vi "ChannelNamingExample.vi"() -> ()   [LabVIEW 2023]
uses:
  <vilib>/DAQmx/read.llb/DAQmx Read (Analog 1D Wfm NChan NSamp).vi
  <vilib>/DAQmx/create/channels.llb/DAQmx Create Channel (AI-Voltage-Basic).vi
  <vilib>/DAQmx/configure/timing.llb/DAQmx Timing (Sample Clock).vi
  <vilib>/DAQmx/miscellaneous.llb/DAQmx Fill In Error Info.vi
panel:
  out "data":waveform(dbl)[](array[waveform])
  out "Waveform Chart":waveform(dbl)[](graph)
  in  "Stop":bool
  in  "Channel Names":string[](array[string])
  in  "Input Channels":tag
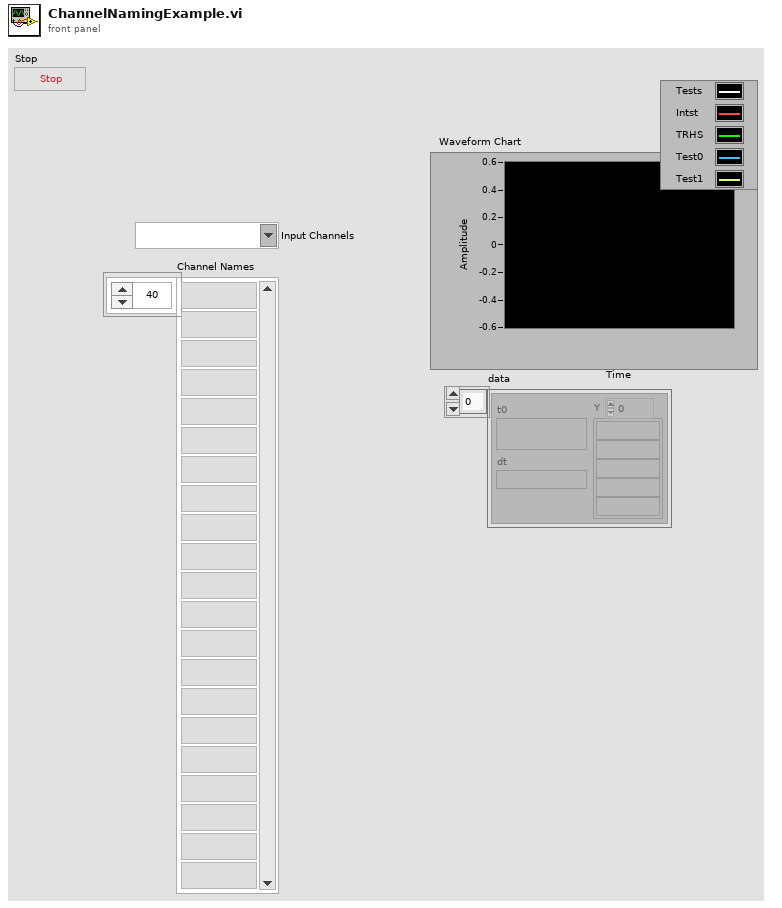
[diagram p1: front panel]
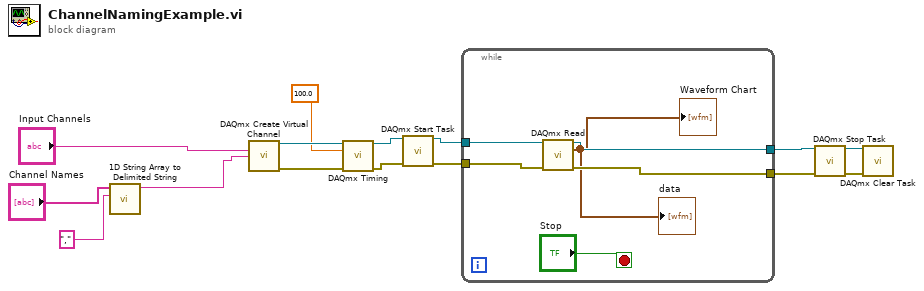
[diagram p0: block diagram]
diagram:
  n1 = call <vilib>:"1D String Array to Delimited String.vi"("delimiter"=",", "string array"="Channel Names") -> ("delimited string"=w12:string)  [unwired: 9 in]
  n2 = call-poly <vilib>:"DAQmx Create Virtual Channel.vi"("physical channels"="Input Channels", "name to assign"=w12) -> ("task out"=w4:refnum<k21>, "error out"=w5:errorcluster)  [unwired: 12 in]
  n3 = call-poly <vilib>:"DAQmx Timing.vi"("task/channels in"=w4, "rate"=100.0, "error in"=w5) -> ("task out"=w2:refnum<k21>, "error out"=w1:errorcluster)  [unwired: 11 in]
  n4 = call <vilib>:"DAQmx Start Task.vi"("task/channels in"=w2, "error in"=w1) -> ("task out"=w11:refnum<k21>, "error out"=w10:errorcluster)  [unwired: 12 in]
  n5 = while {
    tunnel: w11 -> [w20]
    tunnel: w10 -> [w19]
    tunnel: [w18] -> w9
    tunnel: [w17] -> w8
    stop <- "Stop" stop-if-true
    n6 = call-poly <vilib>:"DAQmx Read.vi"("task/channels in"=w20, "error in"=w19) -> ("task out"=w18:refnum<k21>, "data"=→"Waveform Chart" →"data":waveform(dbl)[], "error out"=w17:errorcluster)  [unwired: 11 in]
  }
  n7 = call <vilib>:"DAQmx Stop Task.vi"("task/channels in"=w9, "error in"=w8) -> ("task out"=w7:refnum<k21>, "error out"=w6:errorcluster)  [unwired: 12 in]
  n8 = call <vilib>:"DAQmx Clear Task.vi"("task in"=w7, "error in"=w6) -> ()  [unwired: 13 in, 1 out]
